vi "Heater Auto (Set).vi"(6 "ISOBUS address":T2=-1 caption="ISOBUS address (-1)", 8 "error in":errorcluster, 10 "Heater Auto":string, 11 "Mercury Reference In":T4) -> (0 "error out":errorcluster, 2 "Response":T1, 3 "Mercury Reference Out":T4, 4 "Valid?":T3)   [LabVIEW 2015, in "Mercury iXX.lvlib" / "Control Loop.lvlib"]
doc: "Set the Heater to be in automatic mode or not."
uses:
  Control Loop.lvlib
  Controls/Mercury Reference.ctl
  Controls/Comms Transport Layer.ctl
  Private/Controls/Query Dynamic Reference.ctl
  Controls/Is Valid LED.ctl
  Controls/ISOBus Address.ctl
  Controls/Response String.ctl
  Private/Controls/Command Verbs.ctl
  Mercury iXX.lvlib
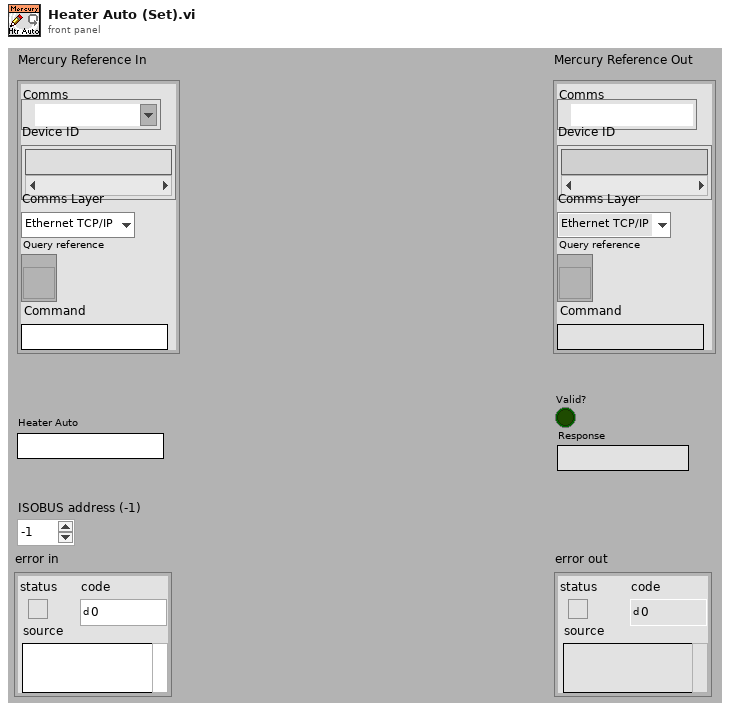
[diagram p1: front panel]
types:
  T1 = typedef "Mercury iXX.lvlib/Response String.ctl" = string
  T2 = typedef "Mercury iXX.lvlib/ISOBus Address.ctl" = i32
  T3 = typedef "Mercury iXX.lvlib/Is Valid LED.ctl" = bool
  T4 = typedef "Mercury iXX.lvlib/Mercury Reference.ctl" = cluster{"Comms":refnum<visa-resource-name>, "Device ID":string[], "Comms Layer":T5, "Command":string, "Query reference":T6}
  T5 = typedef "Mercury iXX.lvlib/Comms Transport Layer.ctl" = enum16{"Ethernet TCP/IP", "USB", "ISOBus - RS-232", "GPIB"}
  T6 = typedef "Mercury iXX.lvlib/Query Dynamic Reference.ctl" = refnum<vi>
  T7 = typedef "Mercury iXX.lvlib/Command Verbs.ctl" = string
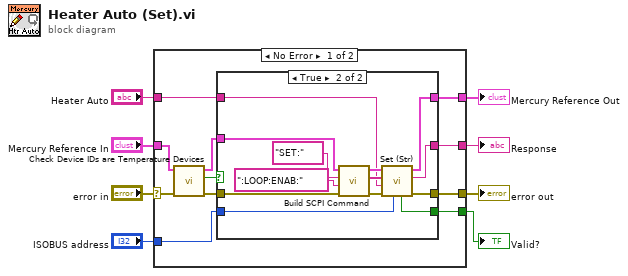
[diagram p0: block diagram]
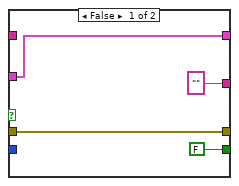
[diagram p2: hidden frame]
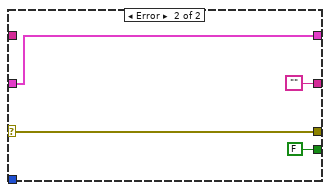
[diagram p3: hidden frame]
diagram:
  n1 = case shown="No Error" "error in" {
    selector: "error in" -> [w15 w39]
    tunnel: "Mercury Reference In" -> [w13 w40]
    tunnel: [w18 w40] -> w5
    tunnel: [w17 w39] -> w2
    tunnel: "ISOBUS address" -> [w19 _]
    tunnel: [w9 ""] -> w4
    tunnel: [w10 FALSE ("Valid?")] -> w3
    tunnel: "Heater Auto" -> [w11 _]
    frame No Error {
      n2 = call "Check Device IDs are Temperature Devices.vi"("error in"=w15, "Mercury Reference In"=w13) -> ("error out"=w14:errorcluster, "Valid?"=w16:bool, "Mercury Reference Out"=w12:T4)  [unwired: 7 out]
      n3 = case shown="True" w16 {
        tunnel: w14 -> [w23 w25]
        tunnel: w19 -> [_ w30]
        tunnel: w12 -> [w22 w24]
        tunnel: [w22 w26] -> w18
        tunnel: [w23 w29] -> w17
        tunnel: w11 -> [_ w31]
        tunnel: [T3 FALSE ("Valid?") w28] -> w10
        tunnel: [T1 "" ("Response") w27] -> w9
        frame False {
        }
        frame True {
          n4 = call "Build SCPI Command.vi"("error in"=w25, "Noun(s)"=":LOOP:ENAB:" ("Command"), "Verb"=T7 "SET:", "Mercury Reference In"=w24) -> ("error out"=w35:errorcluster, "SCPI Message(s)"=w34:string[], "Mercury Reference Out"=w33:T4)  [unwired: 5 out]
          n5 = call "Set (Str).vi"("ISOBUS address"=w30, "error in"=w35, "Command Value (Str)"=w31, "SCPI Message(s)"=w34, "Mercury Reference In"=w33) -> ("error out"=w29:errorcluster, "Response"=w27:T1, "Mercury Reference Out"=w26:T4, "Valid?"=w28:T3)  [unwired: 3 out]
        }
      }
    }
    frame Error {
    }
  }
  "Mercury Reference Out" <- w5
  "error out" <- w2
  "Valid?" <- w3
  "Response" <- w4
